vi "Logical Calculator.vi"(7 "Number 2 (0)":i32, 8 "error in (no error)":errorcluster, 9 "Number 1 (0)":i32, 10 "Operation (0: ADD)":i32(ring) items=["ADD", "OR", "XOR"], 11 "VISA resource name":refnum<visa-resource-name>) -> (0 "error out":errorcluster, 2 "Result":i32, 3 "VISA resource name out":refnum<visa-resource-name>)   [LabVIEW 2015, in "Keithley 2600 Series.lvlib"]
doc: "Performs a bitwise logical operation on two numbers."
uses:
  Keithley 2600 Series.lvlib
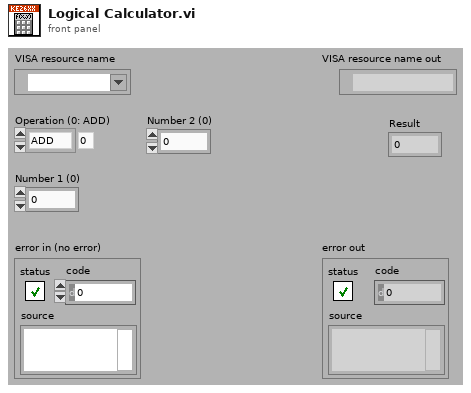
[diagram p1: front panel]
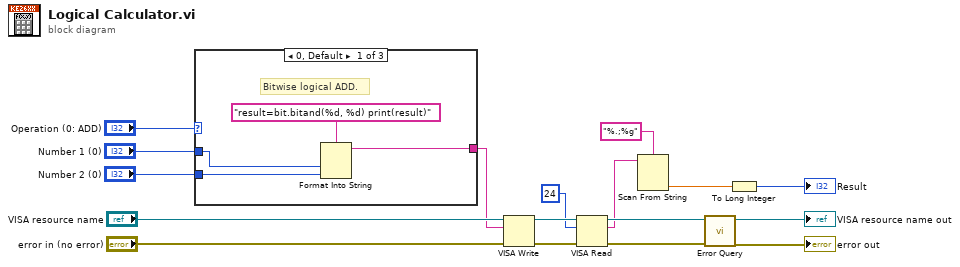
[diagram p0: block diagram]
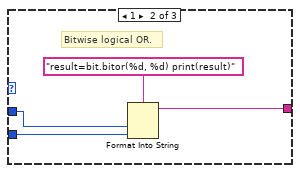
[diagram p2: hidden frame]
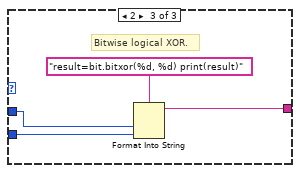
[diagram p3: hidden frame]
diagram:
  n1 = case shown="0, Default" "Operation (0: ADD)" {
    tunnel: "Number 1 (0)" -> [w20 w23 w27]
    tunnel: "Number 2 (0)" -> [w19 w24 w28]
    tunnel: [w18 w22 w26] -> w10
    frame 0, Default {
      # "Bitwise logical ADD."
      n2 = Format Into String(format string="result=bit.bitand(%d, %d) print(result)", w20, w19) -> (resulting string=w18:string)  [unwired: 2 in, 1 out]
    }
    frame 1 {
      # "Bitwise logical OR."
      n3 = Format Into String(format string="result=bit.bitor(%d, %d) print(result)", w23, w24) -> (resulting string=w22:string)  [unwired: 2 in, 1 out]
    }
    frame 2 {
      # "Bitwise logical XOR."
      n4 = Format Into String(format string="result=bit.bitxor(%d, %d) print(result)", w27, w28) -> (resulting string=w26:string)  [unwired: 2 in, 1 out]
    }
  }
  n5 = VISA Write(VISA resource name="VISA resource name", write buffer=w10, error in (no error)="error in (no error)") -> (VISA resource name out=w9:refnum<visa-resource-name>, error out=w8:errorcluster)  [unwired: 1 out]
  n6 = VISA Read(VISA resource name=w9, byte count=u32 24, error in (no error)=w8) -> (VISA resource name out=w7:refnum<visa-resource-name>, read buffer=w4:string, error out=w6:errorcluster)  [unwired: 1 out]
  n7 = Scan From String(format string="%.;%g", input string=w4) -> (output 1=w1:dbl)  [unwired: 3 in, 3 out]
  n8 = call "Error Query.vi"("error in (no error)"=w6, "VISA resource name"=w7) -> ("error out"=→"error out":errorcluster, "VISA resource name out"=→"VISA resource name out":refnum<visa-resource-name>)  [unwired: 6 in, 2 out]
  n9 = To Long Integer(number=w1) -> (32bit integer=→"Result":i32)
